vi "F to K(2D sgl).vi"(1 "F":sgl[][](array[numeric])) -> (0 "K":sgl[][](array[numeric]))   [LabVIEW 2012, in "Temp Converter.lvlib"]
doc: "<B>输入端子C</B>: 输入华氏温度。\n<B>输出端子C</B>: 输出摄氏温度。\n\n公式：F-->C-->K\n创建者：CSXCS_366"
uses:
  Temp Converter.lvlib
  FtoC/F to C (2D sgl).vi
  CtoK/C to K (2D sgl).vi
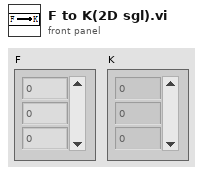
[diagram p1: front panel]
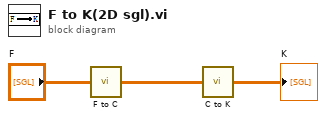
[diagram p0: block diagram]
diagram:
  n1 = call-poly "F to C.vi"("F"="F") -> ("C"=w2:sgl[][])
  n2 = call-poly "C to K.vi"("C"=w2) -> ("K"=→"K":sgl[][])
